vi "read_command.vi"(8 "error in (no error)":errorcluster, 10 "Current Comm. Num.":dbl, 11 "Path":path) -> (0 "error out":errorcluster, 1 "Last Command  Reached":bool, 2 "Next Comm. Num.":dbl, 3 "Command":string)   [LabVIEW 2011]
uses:
  delay_time.vi
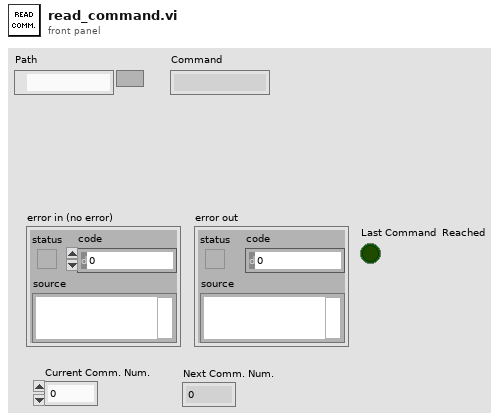
[diagram p1: front panel]
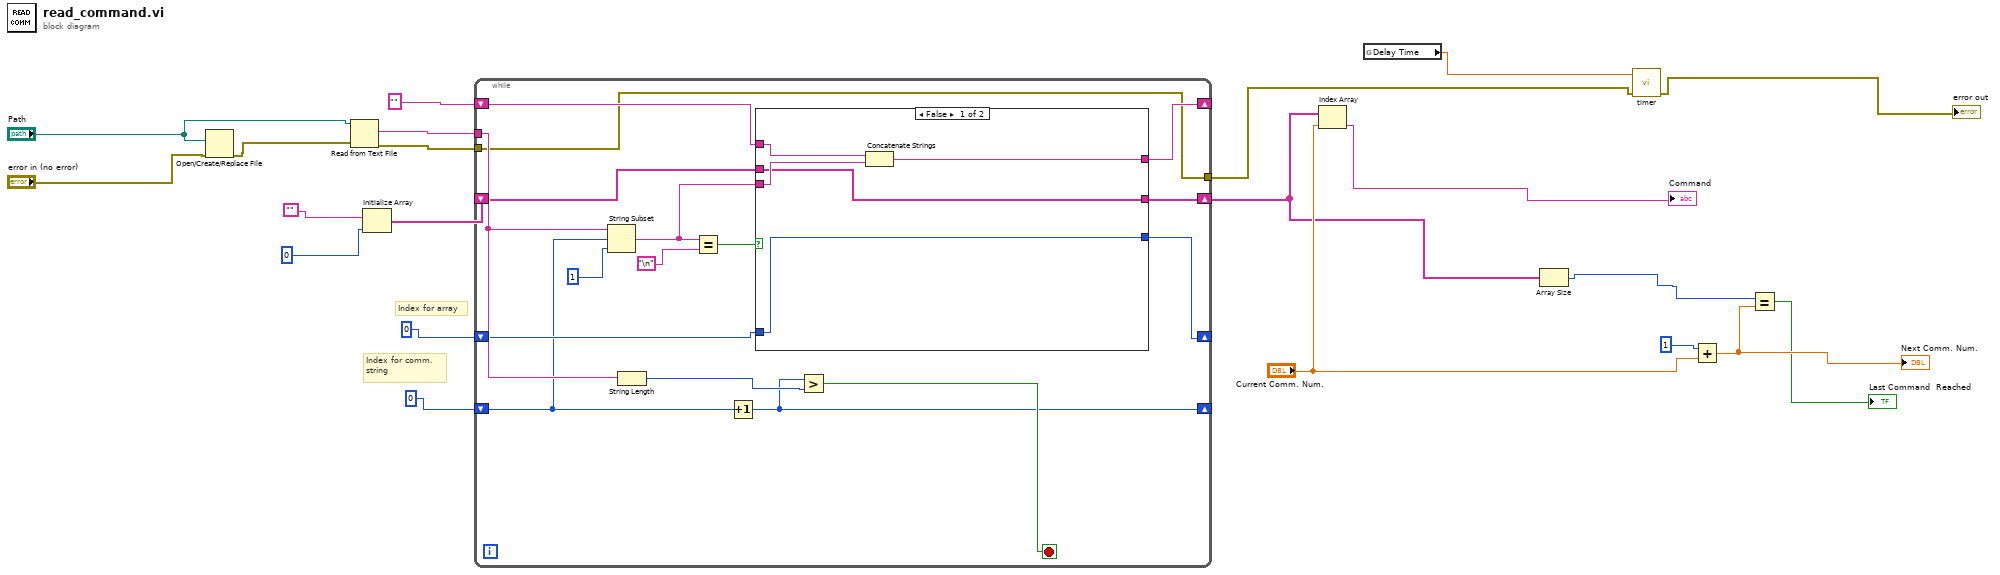
[diagram p0: block diagram]
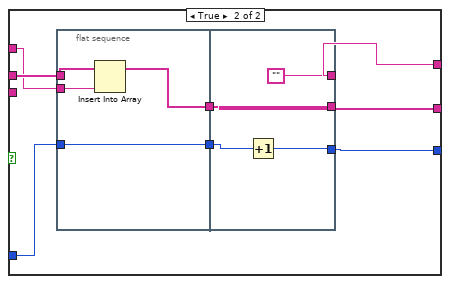
[diagram p2: hidden frame]
diagram:
  # "Index for comm.\nstring"
  # "Index for array"
  n1 = Open/Create/Replace File(file path (use dialog)="Path", error in="error in (no error)") -> (error out=w7:errorcluster)  [unwired: 4 in, 2 out]
  n2 = Read from Text File(file (use dialog)="Path", error in=w7) -> (text=w16:string, error out=w15:errorcluster)  [unwired: 2 in, 2 out]
  n3 = Initialize Array("", 0) -> (w11:string[])
  n4 = while {
    tunnel: w16 -> [w34]
    tunnel: w15 -> [w24]
    shift-right: [w22] -> _
    shift-left: 0 -> [w23]
    shift-right: [w29] -> _
    shift-left: "" -> [w30]
    shift-right: [w27] -> w6
    shift-left: w11 -> [w28]
    shift-right: [w25] -> _
    shift-left: 0 -> [w26]
    tunnel: [w24] -> w3
    stop <- w36 stop-if-true
    n5 = String Subset(string=w34, offset (0)=w23, length (rest)=1) -> (substring=w31:string)
    n6 = String Length(string=w34) -> (length=w37:i32)
    n7 = Equal?(x=w31, y="\n") -> (x = y?=w32:bool)
    n8 = Increment(x=w23) -> (x+1=w22:i32)
    n9 = case shown="False" w32 {
      tunnel: w31 -> [w42 _]
      tunnel: [w41 w46] -> w29
      tunnel: w30 -> [w40 w49]
      tunnel: w28 -> [w39 w50]
      tunnel: [w39 w48] -> w27
      tunnel: w26 -> [w38 w45]
      tunnel: [w38 w43] -> w25
      frame False {
        n10 = Concatenate Strings(w40, w42) -> (w41:string)
      }
      frame True {
        n11 = flat-sequence {
          tunnel: w50 -> [w54]
          tunnel: w49 -> [w53]
          tunnel: [w52] -> w47
          tunnel: w45 -> [w51]
          tunnel: [w51] -> w44
          tunnel: [w58] -> w48
          tunnel: w47 -> [w58]
          tunnel: [""] -> w46
          tunnel: w44 -> [w56]
          tunnel: [w55] -> w43
          frame #0 {
            n12 = Insert Into Array(array=w54, new element=w53) -> (w52:string[])  [unwired: 1 in]
          }
          frame #1 {
            n13 = Increment(x=w56) -> (x+1=w55:i32)
          }
        }
      }
    }
    n14 = Greater?(x=w22, y=w37) -> (0:w36:bool)
  }
  n15 = Index Array(array=w6, index="Current Comm. Num.") -> (element=→"Command":string)
  n16 = global read "delay_time.vi" "Delay Time"() -> (w1:dbl)
  n17 = Array Size(array=w6) -> (size(s)=w4:i32)
  n18 = call "timer.vi"("error in (no error)"=w3, "Delay Time"=w1) -> ("error out"=→"error out":errorcluster)  [unwired: 9 in]
  n19 = Add(x=1, y="Current Comm. Num.") -> (x+y=w18:dbl)
  "Next Comm. Num." <- w18
  n20 = Equal?(x=w4, y=w18) -> (x = y?=→"Last Command  Reached":bool)
